vi "Module.Set Record Parameters.vi"(7 "Samples Per  IOMod Tick":u16=2, 8 "Record Count":u16=3000, 9 "% of Hold Off Time":dbl=10.0, 10 "% of Pre-Trigger Samples":dbl=10.0, 11 "Total Number of Samples":u16=3000) -> (0 "Actual Num of Hold Off Samples":dbl, 1 "Actual Num of Pre Trigger Samples":dbl, 2 "Actual Record Length":u16=3000, 3 "Record Parameters":T1)   [LabVIEW 2012]
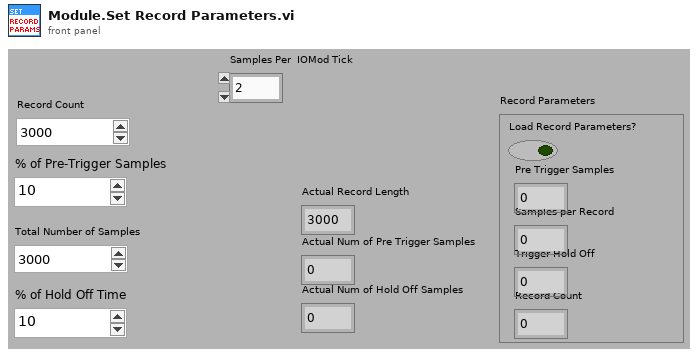
[diagram p1: front panel]
types:
  T1 = cluster{"Load Record Parameters?":bool, "Pre Trigger Samples":u16, "Samples per Record":u16, "Trigger Hold Off":u16, "Record Count":u16}
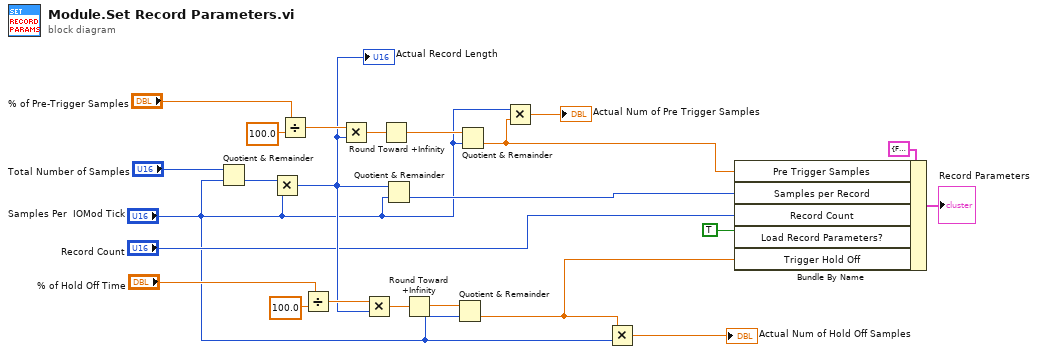
[diagram p0: block diagram]
diagram:
  n1 = Quotient & Remainder(x="Total Number of Samples", y="Samples Per  IOMod Tick") -> (floor(x/y)=w18:u16)  [unwired: 1 out]
  n2 = Multiply(x=w18, y="Samples Per  IOMod Tick") -> (x*y=w8:u16)
  "Actual Record Length" <- w8
  n3 = Divide(x="% of Pre-Trigger Samples", y=100.0) -> (x/y=w22:dbl)
  n4 = Divide(x="% of Hold Off Time", y=100.0) -> (x/y=w11:dbl)
  n5 = Multiply(x=w22, y=w8) -> (x*y=w21:dbl)
  n6 = Multiply(x=w11, y=w8) -> (x*y=w12:dbl)
  n7 = Round Toward +Infinity(x=w21) -> (ceil(x): smallest int >= x=w20:dbl)
  n8 = Quotient & Remainder(x=w8, y="Samples Per  IOMod Tick") -> (floor(x/y)=w13:u16)  [unwired: 1 out]
  n9 = Round Toward +Infinity(x=w12) -> (ceil(x): smallest int >= x=w7:dbl)
  n10 = Quotient & Remainder(x=w7, y="Samples Per  IOMod Tick") -> (floor(x/y)=w1:dbl)  [unwired: 1 out]
  n11 = Quotient & Remainder(x=w20, y="Samples Per  IOMod Tick") -> (floor(x/y)=w16:dbl)  [unwired: 1 out]
  n12 = Multiply(x="Samples Per  IOMod Tick", y=w16) -> (x*y=→"Actual Num of Pre Trigger Samples":dbl)
  n13 = Multiply(x=w1, y="Samples Per  IOMod Tick") -> (x*y=→"Actual Num of Hold Off Samples":dbl)
  n14 = Bundle By Name(cluster=T1 {"Load Record Parameters?"=FALSE, "Pre Trigger Samples"=0, "Samples per Record"=0, "Trigger Hold Off"=0, "Record Count"=0} ("Record Parameters"), "Pre Trigger Samples"=w16, "Samples per Record"=w13, "Record Count"="Record Count", "Load Record Parameters?"=TRUE, "Trigger Hold Off"=w1) -> (→"Record Parameters":T1)
